vi "LVtoJSON-DBUpdate.vi"(0 "Table":string="Inventory", 1 "Update All":bool, 2 "SQL Query Statement":string, 3 "Column Number":i32, 5 "SQL Statement":string, 7 "Columns":string[](array[string]), 11 "error in":errorcluster, 12 "Payload":string="Inventory", 14 "Datatype":i32) -> (4 "Output JSON Object":string, 15 "error out":errorcluster)   [LabVIEW 2014]
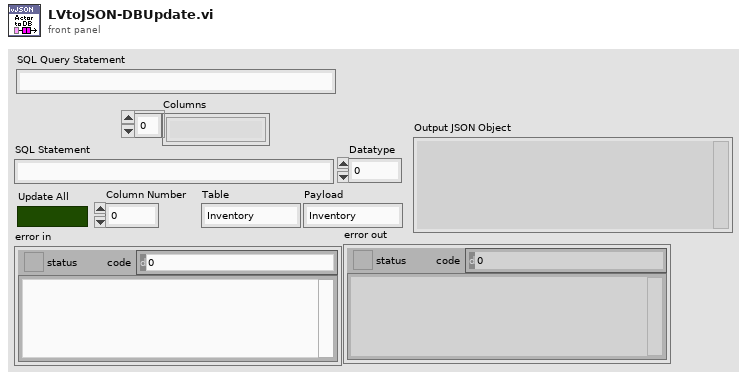
[diagram p1: front panel]
types:
  T1 = cluster{"Table":string, "SQL Statement":string, "Update All":bool, "Payload":string, "Column Number":i32, "Datatype":i32, "SQL Query Statement":string, "Columns":string}
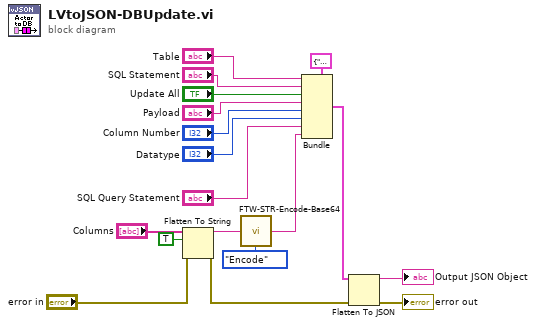
[diagram p0: block diagram]
diagram:
  n1 = Flatten To String(anything="Columns", prepend array or string size? (T)=TRUE, error in (no error)="error in") -> (data string=w7:string, error out=w4:errorcluster)  [unwired: 1 in, 1 out]
  n2 = call "FTW-STR-Encode-Base64.vi"("Input"=w7, "Direction"=enum16{"Encode", "Decode"}."Encode") -> ("Output"=w1:string)
  n3 = Bundle(cluster=T1 {"Table"="", "SQL Statement"="", "Update All"=FALSE, "Payload"="", "Column Number"=0, "Datatype"=0, "SQL Query Statement"="", "Columns"=""} ("output cluster"), "Table"="Table", "SQL Statement"="SQL Statement", "Update All"="Update All", "Payload"="Payload", "Column Number"="Column Number", "Datatype"="Datatype", "SQL Query Statement"="SQL Query Statement", "Columns"=w1) -> (w13:T1)
  n4 = Flatten To JSON(anything=w13, error in (no error)=w4) -> (JSON string=→"Output JSON Object":string, 11:→"error out":errorcluster)  [unwired: 1 in]
